vi "SectionA04_Week4_Stus.vi"() -> ()   [LabVIEW 2013]
uses:
  <vilib>/Analysis/3filter.llb/Filter Passband Type.ctl
  <vilib>/Analysis/3filter.llb/Butterworth Filter (DBL).vi
  <vilib>/Analysis/NI_AALBase.lvlib
panel:
  out "Processed Signal":dbl[](graph)
  in  "?":bool
  in  "Signal Processing":T1(radio)
  in  "Cut off Frequency":dbl(slide) scale=0.0..0.5
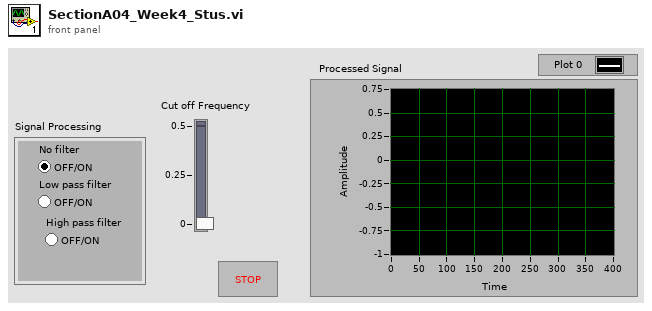
[diagram p1: front panel]
types:
  T1 = enum32{"No filter", "Low pass filter", "High pass filter"}
  T2 = typedef "NI_AALBase.lvlib/Filter Passband Type.ctl" = enum32{"Lowpass", "Highpass", "Bandpass", "Bandstop"}
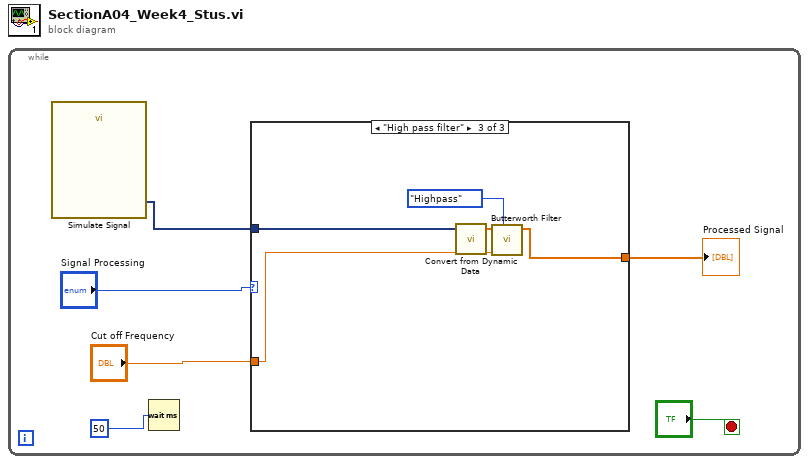
[diagram p0: block diagram]
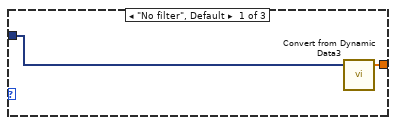
[diagram p2: hidden frame]
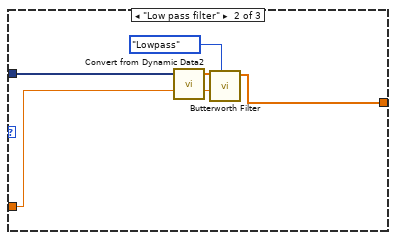
[diagram p3: hidden frame]
diagram:
  n1 = while {
    stop <- "?" stop-if-true
    n2 = call "Simulate Signal"() -> ("Sine with Uniform Noise"=w2:dynamicdata)  [unwired: 14 in, 1 out]
    n3 = Wait (ms)(milliseconds to wait=50) -> ()  [unwired: 1 out]
    n4 = case shown="\"High pass filter\"" "Signal Processing" {
      tunnel: "Cut off Frequency" -> [_ w11 w18]
      tunnel: w2 -> [w8 w13 w17]
      tunnel: [w7 w10 w15] -> w1
      frame "No filter", Default {
        n5 = call "Convert from Dynamic Data3"("Dynamic Data Type"=w8) -> ("Array"=w7:dbl[])  [unwired: 3 in]
      }
      frame "Low pass filter" {
        n6 = call "Convert from Dynamic Data2"("Dynamic Data Type"=w13) -> ("Array"=w12:dbl[])  [unwired: 3 in]
        n7 = call-poly <vilib>:"Butterworth Filter.vi"("filter type"=Filter_Passband_Type."Lowpass", "high cutoff freq: fh"=w11, "X"=w12) -> ("Filtered X"=w10:dbl[])  [unwired: 5 in, 1 out]
      }
      frame "High pass filter" {
        n8 = call "Convert from Dynamic Data"("Dynamic Data Type"=w17) -> ("Array"=w16:dbl[])  [unwired: 3 in]
        n9 = call-poly <vilib>:"Butterworth Filter.vi"("filter type"=Filter_Passband_Type."Highpass", "low cutoff freq: fl"=w18, "X"=w16) -> ("Filtered X"=w15:dbl[])  [unwired: 5 in, 1 out]
      }
    }
    "Processed Signal" <- w1
  }
